vi "CAPTH-Load Data.vi"(0 "Path":path) -> (4 "graph":cluster{dbl[], dbl[]}[](graph), 8 "data":T1(array[cluster]))   [LabVIEW 2020]
uses:
  <vilib>/Analysis/polynomials.llb/Unique Numbers and Multiplicity (DBL).vi
  <vilib>/Analysis/NI_AALPro.lvlib
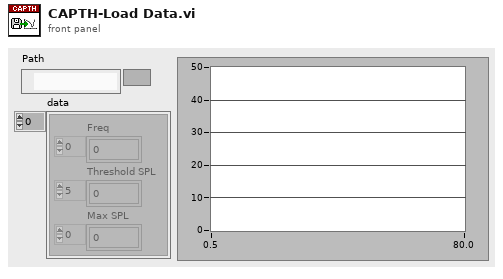
[diagram p1: front panel]
types:
  T1 = cluster{"Freq":dbl[], "Threshold SPL":dbl[], "Max SPL":dbl[]}[]
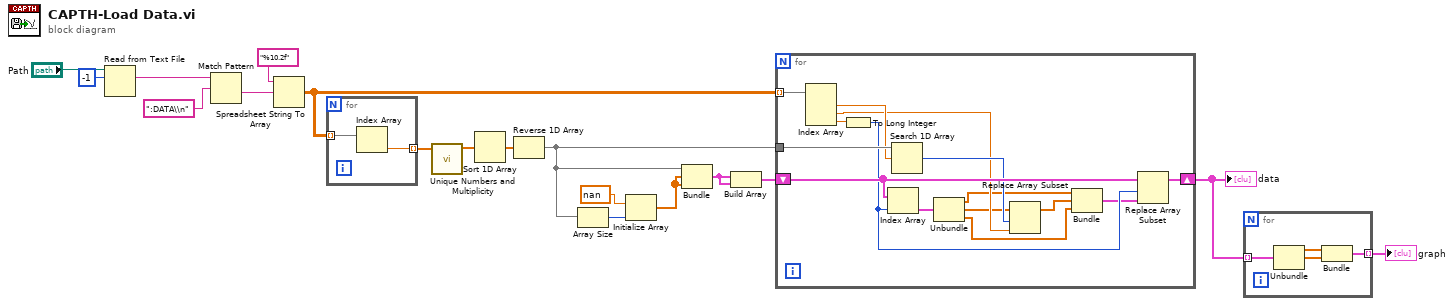
[diagram p0: block diagram]
diagram:
  n1 = Read from Text File(file (use dialog)="Path", count=-1) -> (text=w15:string)  [unwired: 2 in, 3 out]
  n2 = Match Pattern(string=w15, regular expression=":DATA\\n") -> (after substring=w14:string)  [unwired: 1 in, 3 out]
  n3 = Spreadsheet String To Array(format string="%10.2f", spreadsheet string=w14) -> (array=w7:dbl[][])  [unwired: 2 in]
  n4 = for {
    tunnel: w7 -> [w20] mode=indexing
    tunnel: [w19] -> w12 mode=indexing
    n5 = Index Array(array=w20) -> (element=w19:dbl)  [unwired: 1 in]
  }
  n6 = call-poly <vilib>:"Unique Numbers and Multiplicity.vi"("Numbers"=w12) -> ("Unique Numbers"=w8:dbl[])  [unwired: 8 in, 2 out]
  n7 = Sort 1D Array(array=w8) -> (sorted array=w6:dbl[])
  n8 = Reverse 1D Array(array=w6) -> (reversed array=w1:dbl[])
  n9 = Array Size(array=w1) -> (size(s)=w11:i32)
  n10 = Initialize Array(nan ("element"), w11) -> (w4:dbl[])
  n11 = Bundle(w1, w4, w4) -> (w9:cluster{dbl[], dbl[], dbl[]})  [unwired: 1 in]
  n12 = Build Array(w9, w9) -> (w5:cluster{dbl[], dbl[], dbl[]}[])
  n13 = for {
    tunnel: w7 -> [w35] mode=indexing
    shift-right: [w31] -> w3
    shift-left: w5 -> [w30]
    tunnel: w1 -> [w33]
    n14 = Index Array(array=w35) -> (element #1=w32:dbl, element #2=w26:dbl, element #3=w34:dbl)  [unwired: 3 in]
    n15 = To Long Integer(number=w34) -> (32bit integer=w29:i32)
    n16 = Index Array(array=w30, index=w29) -> (element=w28:cluster{dbl[], dbl[], dbl[]})
    n17 = Search 1D Array(1D array=w33, element=w32) -> (index of element=w27:i32)  [unwired: 1 in]
    n18 = Unbundle(w28) -> (w25:dbl[], w23:dbl[], w21:dbl[])
    n19 = Replace Array Subset(array=w23, new element=w26, index=w27) -> (w22:dbl[])
    n20 = Bundle(w25, w22, w21) -> (w24:cluster{dbl[], dbl[], dbl[]})  [unwired: 1 in]
    n21 = Replace Array Subset(array=w30, new element=w24, index=w29) -> (w31:cluster{dbl[], dbl[], dbl[]}[])
  }
  "data" <- w3
  n22 = for {
    tunnel: w3 -> [w39] mode=indexing
    tunnel: [w36] -> w2 mode=indexing
    n23 = Unbundle(w39) -> (w38:dbl[], w37:dbl[])  [unwired: 1 out]
    n24 = Bundle(w38, w37) -> (w36:cluster{dbl[], dbl[]})  [unwired: 1 in]
  }
  "graph" <- w2
